vi "bang-bang-ElevatorSim_example.vi"() -> ()   [LabVIEW 2019]
uses:
  <vilib>/Rock Robotics/WPI/ThirdParty/JAS_Junk/TrajLib/Trajectory_Library.lvlib
  <vilib>/Analysis/Matrix/Datatypes/RealMatrix.ctl
  <vilib>/Analysis/Matrix/NI_Matrix.lvlib
  <vilib>/Rock Robotics/WPI/ThirdParty/JAS_Junk/TrajLib/LINEAR_SYSTEM.ctl
  <vilib>/Rock Robotics/WPI/ThirdParty/JAS_Junk/TrajLib/DCMOTOR.CTL
  <vilib>/Rock Robotics/WPI/ThirdParty/JAS_Junk/TrajLib/LINEAR_QUADRATIC_REGULATOR.ctl
  <vilib>/Rock Robotics/WPI/ThirdParty/JAS_Junk/TrajLib/KALMAN_FILTER.ctl
  <vilib>/Rock Robotics/WPI/ThirdParty/JAS_Junk/TrajLib/LINEAR_PLANT_INV_FF.ctl
  <vilib>/Rock Robotics/WPI/ThirdParty/JAS_Junk/TrajLib/LINEAR_SYSTEM_LOOP.ctl
  <vilib>/Rock Robotics/WPI/ThirdParty/JAS_Junk/TrajLib/LINEAR_SYSTEM_SIM.ctl
  <vilib>/Rock Robotics/WPI/ThirdParty/JAS_Junk/TrajLib/ELEVATOR_SIM.ctl
panel:
  in  "Tab Control":T1(tab)
  in  "Turn Motor Off":bool
  in  "Use Bang Bang":bool=TRUE
  out "Battery Voltage":dbl format="%20.3f"
  out "CO Chart":cluster{dbl, "Voltage":dbl}(graph)
  in  "GO UP":bool
  out "Elevator\nHeight \nSetpoint(SP)":dbl(slide) scale=-1.0..6.0
  out "Height":dbl format="%20.3f"
  out "Cor Err":bool
  out "Kalman Filtered\nHeight":dbl format="%20.3f"
  out "PV Chart":T2(graph)
  out "Predict Err":bool
  out "Motor Volt Dmd (CO)":dbl format="%20.3f"
  out "At Top":bool
  out "At Bottom":bool
  out "Motor Amps":dbl format="%20.3f"
  out "Elevator Motor":T3 {"Jr_KgM2" format="%13.5p"; "L_H" format="%13.5p"; "Kt_NMPerAmp" format="%13.5p"; "KvINV_RadPerSecPerVolt" format="%13.5p"; "R_Ohms" format="%13.5p"; "FreeSpeed_RadPerSec" format="%13.5p"; "FreeCurrent_Amps" format="%13.5p"; "StallCurrent_Amps" format="%13.5p"; "StallTorque_NM" format="%13.5p"; "nominalVoltage_Volts" format="%13.5p"}
  out "m_Elevator":T4
  out "Elevator Simulaation":T6 {"GearBox"."Jr_KgM2" format="%13.5p"; "GearBox"."L_H" format="%13.5p"; "GearBox"."Kt_NMPerAmp" format="%13.5p"; "GearBox"."KvINV_RadPerSecPerVolt" format="%13.5p"; "GearBox"."R_Ohms" format="%13.5p"; "GearBox"."FreeSpeed_RadPerSec" format="%13.5p"; "GearBox"."FreeCurrent_Amps" format="%13.5p"; "GearBox"."StallCurrent_Amps" format="%13.5p"; "GearBox"."StallTorque_NM" format="%13.5p"; "GearBox"."nominalVoltage_Volts" format="%13.5p"}
  out "KalmanFilter":T8
  out "Kalman Error":errorcluster
  out "LinearQuadraticRegulator":T9
  out "LQR Error":bool
  out "Linear System Loop":T10
  out "LinSysLoop_Error":bool
  # "THIS IS A SAMPLE  -- THERE ARE BETTER WAYS TO CONTROL THIS OTHER THAN BANG-BANG"
  # "<States,States>"
  # "<States,Inputs>"
  # "<Outputs,States>"
  # "<Outputs,Inputs>"
  # "<States, 1>"
  # "<Outputs, 1>"
  # "<Inputs, 1>"
  # "<Outputs, 1>"
  # "<States,States>"
  # "<States,Inputs>"
  # "<Outputs,States>"
  # "<Outputs,Inputs>"
  # "Steady State Gain  \n<States,Outputs>"
  # "State Estimate <Statess,1>"
  # "<States,States>"
  # "<States,Inputs>"
  # "<Outputs,States>"
  # "<Outputs,Inputs>"
  # "Ref State <States,1>"
  # "Comp and capped \noutput <Inputs,1>"
  # "Controller gain\n<Inputs,States>"
  # "<States,1>"
  # "<FUTURE --- CLAMP TYPE -- For now\nuse Normalize>"
  # "Steady State Gain  \n<States,Outputs>"
  # "State Estimate <Statess,1>"
  # "<States,States>"
  # "<States,Inputs>"
  # "<Outputs,States>"
  # "<Outputs,Inputs>"
  # "<States,1>"
  # "<Inputs,1>"
  # "<States,Inputs>"
  # "<States,States>"
  # "Ref State <States,1>"
  # "Comp and capped \noutput <Inputs,1>"
  # "Controller gain\n<Inputs,States>"
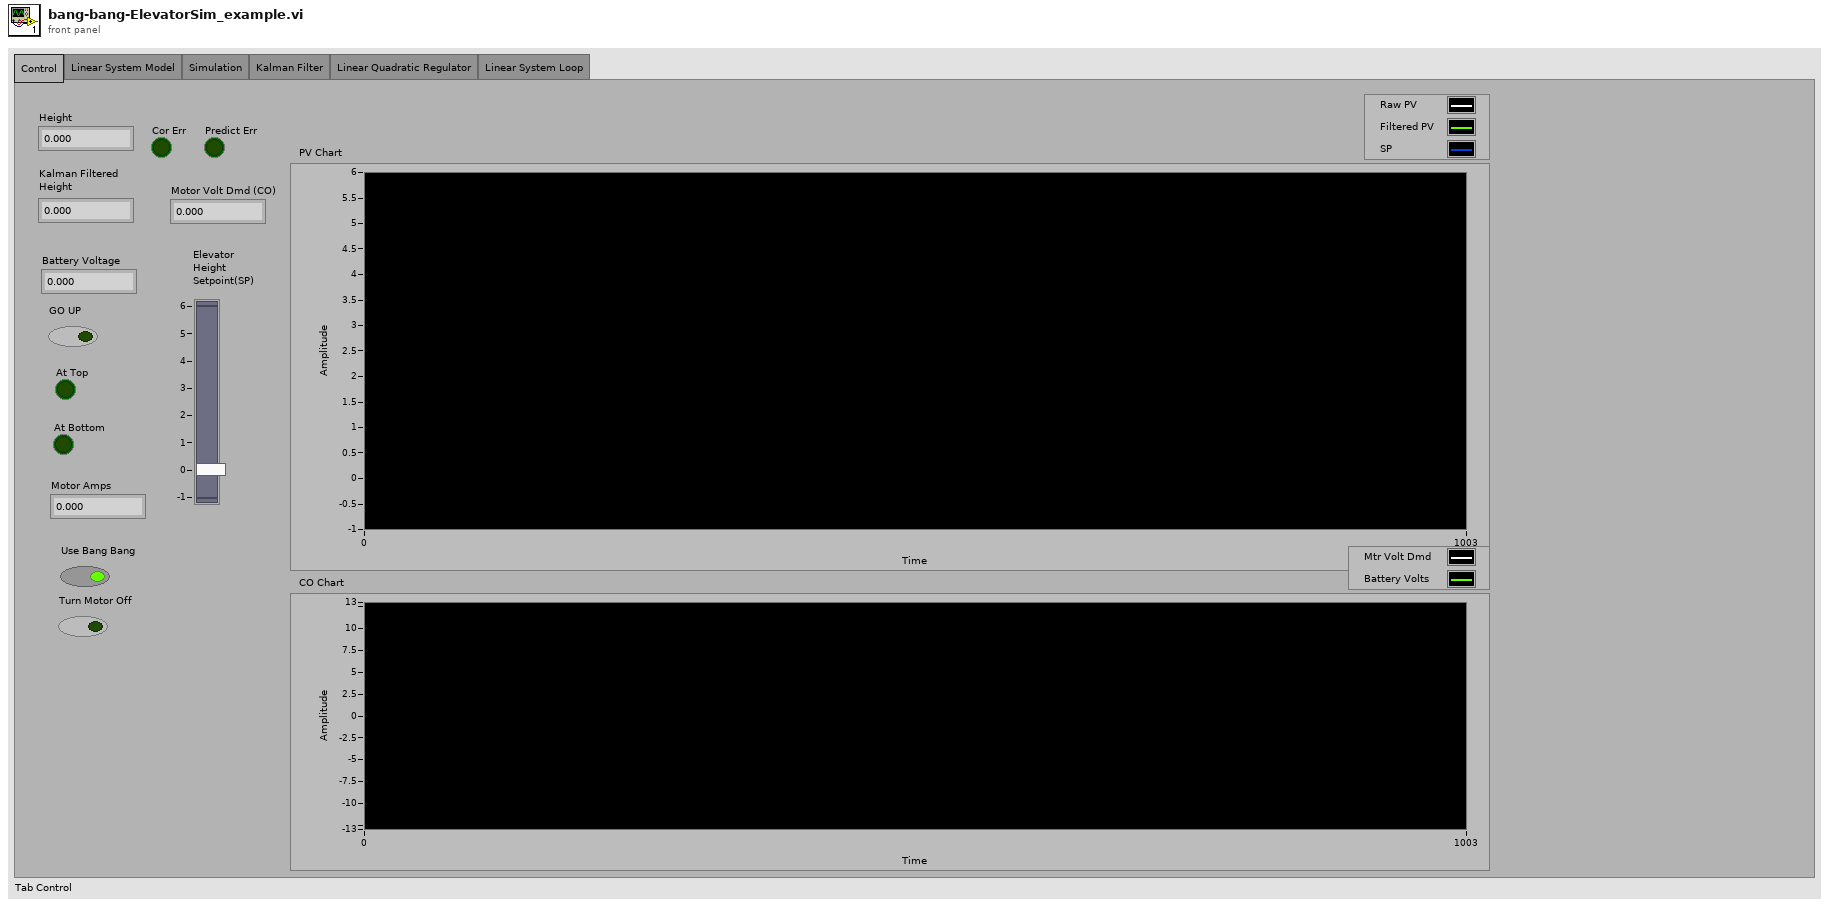
[diagram p1: front panel]
types:
  T1 = enum32{"Control", "Linear System Model", "Simulation", "Kalman Filter", "Linear Quadratic Regulator", "Linear System Loop"}
  T2 = cluster{"upper limit":dbl, "Real Matrix Element":dbl, "Real Matrix Element":dbl}
  T3 = typedef "Trajectory_Library.lvlib/DCMOTOR.CTL" = cluster{"nominalVoltage_Volts":dbl, "StallTorque_NM":dbl, "StallCurrent_Amps":dbl, "FreeCurrent_Amps":dbl, "FreeSpeed_RadPerSec":dbl, "R_Ohms":dbl, "KvINV_RadPerSecPerVolt":dbl, "Kt_NMPerAmp":dbl, "L_H":dbl, "Jr_KgM2":dbl}
  T4 = typedef "Trajectory_Library.lvlib/LINEAR_SYSTEM.ctl" = cluster{"m_A":T5, "m_B":T5, "m_C":T5, "m_D":T5, "States":i32, "Inputs":i32, "Outputs":i32}
  T5 = typedef "NI_Matrix.lvlib/RealMatrix.ctl" = dbl[][]
  T6 = typedef "Trajectory_Library.lvlib/ELEVATOR_SIM.ctl" = cluster{"LinearSystemSim":T7, "GearBox":T3, "Gearing":dbl, "DrumRadius_M":dbl, "MinHeight_M":dbl, "MaxHeight_M":dbl, "CarriageMass_Kg":dbl}
  T7 = typedef "Trajectory_Library.lvlib/LINEAR_SYSTEM_SIM.ctl" = cluster{"m_Plant":T4, "m_X":T5, "m_Y":T5, "m_U":T5, "MeasureStdDev":T5}
  T8 = typedef "Trajectory_Library.lvlib/KALMAN_FILTER.ctl" = cluster{"m_K":T5, "m_xHat":T5, "States":i32, "Outputs":i32, "m_Plant":T4}
  T9 = typedef "Trajectory_Library.lvlib/LINEAR_QUADRATIC_REGULATOR.ctl" = cluster{"m_r":T5, "m_U":T5, "m_K":T5, "States":i32, "Inputs":i32}
  T10 = typedef "Trajectory_Library.lvlib/LINEAR_SYSTEM_LOOP.ctl" = cluster{"Controller":T9, "FeedForward":T11, "Observer":T8, "Next_R":T5, "Clamp Max":T5}
  T11 = typedef "Trajectory_Library.lvlib/LINEAR_PLANT_INV_FF.ctl" = cluster{"m_R":T5, "m_Uff":T5, "m_B":T5, "m_A":T5, "States":i32, "Inputs":i32}
  T12 = cluster{"Position_Meters":dbl, "Real Matrix Element":dbl, "Real Matrix Element":dbl}
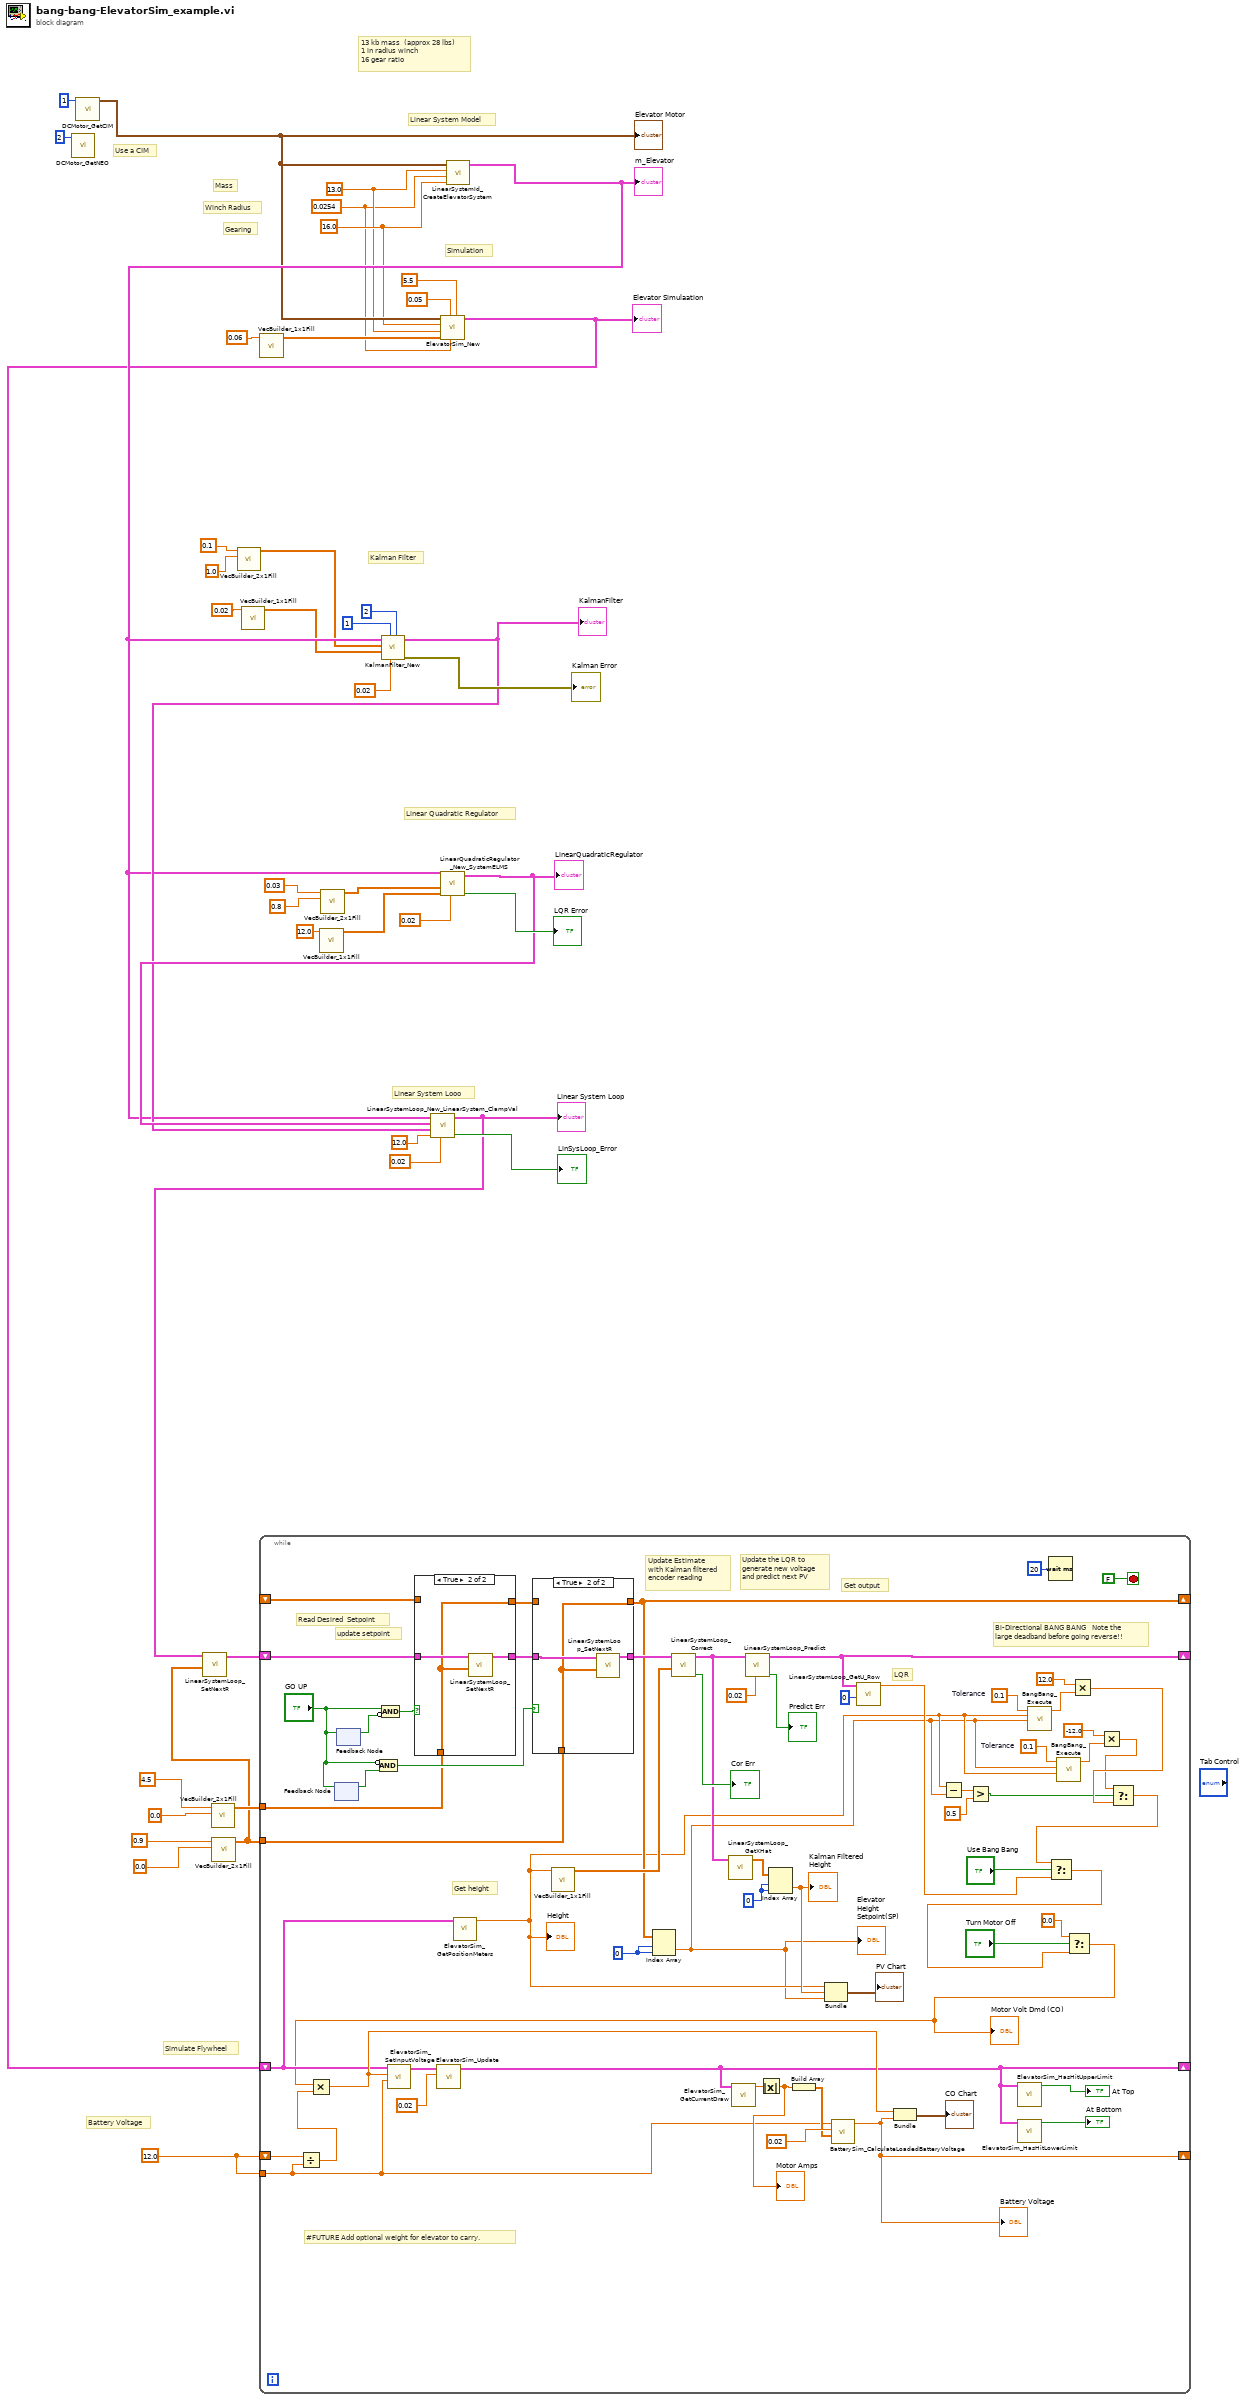
[diagram p0: block diagram]
diagram:
  w26 = 16.0 ("G")
  w24 = 0.0254 ("radiusMeters")
  w25 = 13.0 ("massKg")
  w34 = 12.0
  # "Linear System Looo"
  # "Linear Quadratic Regulator"
  # "Kalman Filter"
  # "Simulation"
  # "Linear System Model"
  # "Mass"
  # "Winch Radius"
  # "Simulate Flywheel"
  # "13 kb mass  (approx 28 lbs)\n1 in radius winch\n16 gear ratio"
  # "Gearing"
  # "Use a CIM"
  # "Battery Voltage"
  n1 = call <vilib>:"DCMotor_GetNEO.vi"("Num Motors"=2) -> ()  [unwired: 10 in, 1 out]
  n2 = call <vilib>:"DCMotor_GetCIM.vi"("Num Motors"=1) -> ("DCMOTOR"=w31:T3)  [unwired: 10 in]
  "Elevator Motor" <- w31
  n3 = call <vilib>:"VecBuilder_2x1Fill.vi"("R1"=0.0, "R0"=4.5 ("RotationsPerMinute")) -> ("output matrix"=w6:T5)  [unwired: 9 in]
  n4 = call <vilib>:"VecBuilder_2x1Fill.vi"("R1"=0.0, "R0"=0.9 ("R0_C0")) -> ("output matrix"=w1:T5)  [unwired: 9 in]
  n5 = call <vilib>:"VecBuilder_2x1Fill.vi"("R1"=1.0, "R0"=0.1 ("R0_C0")) -> ("output matrix"=w17:T5)  [unwired: 9 in]
  n6 = call <vilib>:"VecBuilder_1x1Fill.vi"("R0_C0"=0.02) -> ("output matrix"=w16:T5)  [unwired: 10 in]
  n7 = call <vilib>:"VecBuilder_1x1Fill.vi"("R0_C0"=0.06) -> ("output matrix"=w27:T5)  [unwired: 10 in]
  n8 = call <vilib>:"VecBuilder_1x1Fill.vi"("R0_C0"=12.0) -> ("output matrix"=w10:T5)  [unwired: 10 in]
  n9 = call <vilib>:"VecBuilder_2x1Fill.vi"("R1"=0.8 ("R0_C0"), "R0"=0.03 ("R0_C0")) -> ("output matrix"=w12:T5)  [unwired: 9 in]
  n10 = call <vilib>:"ElevatorSim_New.vi"("MaxHeight_Meters"=5.5, "DrumRadius_Meters"=w24, "MinHeight_Meters"=0.05, "MeasurementStdDev"=w27, "CarriageMass_Kg"=w25, "Gearing"=w26, "GearBox"=w31) -> ("ElevatorSim"=w30:T6)  [unwired: 3 in, 1 out]
  "Elevator Simulaation" <- w30
  n11 = call <vilib>:"LinearSystemId_CreateElevatorSystem.vi"("G"=w26, "radiusMeters"=w24, "massKg"=w25, "DCMOTOR"=w31) -> ("Linearsystem"=w32:T4)  [unwired: 6 in, 1 out]
  "m_Elevator" <- w32
  n12 = call <vilib>:"KalmanFilter_New.vi"("States"=2, "dt_Seconds"=0.02, "Outputs"=1, "MeasurementStdDevs"=w16, "StateStdDevs"=w17, "Plant"=w32) -> ("Error"=→"Kalman Error":errorcluster, "KalmanFilter"=w38:T8)  [unwired: 4 in]
  "KalmanFilter" <- w38
  n13 = call <vilib>:"LinearQuadraticRegulator_New_SystemELMS.vi"("dt_Seconds"=0.02, "Relms"=w10, "Qelms"=w12, "LINEARSYSTEM"=w32) -> ("Error"=→"LQR Error":bool, "LinearQuadraticRegulator"=w39:T9)  [unwired: 6 in]
  "LinearQuadraticRegulator" <- w39
  n14 = call <vilib>:"LinearSystemLoop_New_LinearSystem_ClampVal.vi"("dT_Seconds"=0.02, "Max_Voltage"=12.0, "Observer"=w38, "Controller"=w39, "Plant"=w32) -> ("Error"=→"LinSysLoop_Error":bool, "Linear System Loop"=w2:T10)  [unwired: 5 in]
  "Linear System Loop" <- w2
  n15 = call <vilib>:"LinearSystemLoop_SetNextR.vi"("R"=w1, "input inear System Loop"=w2) -> ("out Linear System Loop"=w3:T10)  [unwired: 8 in, 1 out]
  n16 = while {
    shift-right: [w70] -> _
    shift-left: w3 -> [w98]
    tunnel: w6 -> [w96]
    tunnel: w1 -> [w95]
    shift-right: [w69] -> _
    shift-left: w30 -> [w64]
    shift-right: [w79] -> _
    shift-left: _ -> [w80]
    shift-right: [w72] -> _
    shift-left: w34 -> [w77]
    tunnel: w34 -> [w63]
    stop <- FALSE stop-if-true
    w53 = 0.1  # Tolerance
    w59 = 0.1  # Tolerance
    w78 = 0 ("index (row)")
    w91 = 0 ("index (row)")
    # "Bi-Directional BANG BANG   Note the\nlarge deadband before going reverse!!"
    # "LQR"
    # "Get height"
    # "#FUTURE Add optional weight for elevator to carry."
    # "Get output"
    # "Update the LQR to \ngenerate new voltage\nand predict next PV"
    # "update setpoint"
    # "Read Desired  Setpoint"
    # "Update Estimate\nwith Kalman filtered\nencoder reading"
    n17 = Divide(x=w77, y=w63) -> (x/y=w76:dbl)
    n18 = feedback #1() -> (w102:bool)  [unwired: 1 in]
    n19 = feedback-in #1("GO UP") -> ()
    n20 = feedback-in #2("GO UP") -> ()
    n21 = feedback #2() -> (w103:bool)  [unwired: 1 in]
    n22 = Compound Arithmetic op=AND(invert "GO UP", w102) -> (w99:bool)
    n23 = Compound Arithmetic op=AND("GO UP", invert w103) -> (w100:bool)
    n24 = case shown="True" w100 {
      tunnel: w98 -> [w112 w114]
      tunnel: [w112 w115] -> w97
      tunnel: w96 -> [_ w113]
      tunnel: [w111 w113] -> w81
      tunnel: w80 -> [w111 _]
      frame False {
      }
      frame True {
        n25 = call <vilib>:"LinearSystemLoop_SetNextR.vi"("R"=w113, "input inear System Loop"=w114) -> ("out Linear System Loop"=w115:T10)  [unwired: 8 in, 1 out]
      }
    }
    n26 = call <vilib>:"ElevatorSim_GetPositionMeters.vi"("ElevatorSim"=w64) -> ("Position_Meters"=w50:dbl)  [unwired: 10 in]
    "Height" <- w50
    n27 = case shown="True" w99 {
      tunnel: w97 -> [w107 w109]
      tunnel: [w107 w110] -> w94
      tunnel: w95 -> [_ w108]
      tunnel: w81 -> [w106 _]
      tunnel: [w106 w108] -> w79
      frame False {
      }
      frame True {
        n28 = call <vilib>:"LinearSystemLoop_SetNextR.vi"("R"=w108, "input inear System Loop"=w109) -> ("out Linear System Loop"=w110:T10)  [unwired: 8 in, 1 out]
      }
    }
    n29 = call <vilib>:"VecBuilder_1x1Fill.vi"("R0_C0"=w50) -> ("output matrix"=w93:T5)  [unwired: 10 in]
    n30 = Index Array(array=w79, index (row)=w78, index (col)=w78) -> (element=w49:dbl)
    "Elevator\nHeight \nSetpoint(SP)" <- w49
    n31 = call <vilib>:"LinearSystemLoop_Correct.vi"("Y"=w93, "input inear System Loop"=w94) -> ("Error"=→"Cor Err":bool, "out Linear System Loop"=w87:T10)  [unwired: 8 in]
    n32 = call <vilib>:"LinearSystemLoop_GetXHat.vi"("input inear System Loop"=w87) -> ("XHat"=w90:T5)  [unwired: 10 in]
    n33 = call <vilib>:"LinearSystemLoop_Predict.vi"("dT_Seconds"=0.02, "input inear System Loop"=w87) -> ("Error"=→"Predict Err":bool, "out Linear System Loop"=w70:T10)  [unwired: 8 in]
    n34 = Index Array(array=w90, index (row)=w91, index (col)=w91) -> (element=w89:dbl)
    "Kalman Filtered\nHeight" <- w89
    n35 = Bundle("Position_Meters"=w50, "Real Matrix Element"=w89, "Real Matrix Element"=w49) -> (→"PV Chart":T12)  [unwired: 1 in]
    n36 = call <vilib>:"LinearSystemLoop_GetU_Row.vi"("Row"=0, "input inear System Loop"=w70) -> ("U"=w55:dbl)  [unwired: 9 in]
    n37 = Subtract(x=w50, y=w49) -> (x-y=w48:dbl)
    n38 = Greater?(x=w48, y=0.5) -> (0:w43:bool)
    n39 = call <vilib>:"BangBang_Execute.vi"("Setpoint"=w49, "Measurment"=w50, "Tolerance"=w59) -> ("ControlOutput"=w58:dbl)  [unwired: 6 in, 2 out]
    n40 = Wait (ms)(milliseconds to wait=u32 20) -> ()  [unwired: 1 out]
    n41 = call <vilib>:"BangBang_Execute.vi"("Setpoint"=w50, "Measurment"=w49, "Tolerance"=w53) -> ("ControlOutput"=w52:dbl)  [unwired: 6 in, 2 out]
    n42 = Multiply(x=12.0, y=w58) -> (x*y=w46:dbl)
    n43 = Multiply(x=-12.0, y=w52) -> (x*y=w44:dbl)
    n44 = Select(t=w44, s=w43, f=w46) -> (s? t:f=w45:dbl)
    n45 = Select(t=w45, s="Use Bang Bang", f=w55) -> (s? t:f=w54:dbl)
    n46 = Select(t=0.0, s="Turn Motor Off", f=w54) -> (s? t:f=w60:dbl)
    "Motor Volt Dmd (CO)" <- w60
    n47 = Multiply(x=w60, y=w76) -> (x*y=w71:dbl)
    n48 = call <vilib>:"ElevatorSim_SetInputVoltage.vi"("Battery_Volts"=w63, "Input_Voltage"=w71, "in ElevatorSim"=w64) -> ("out ElevatorSim"=w83:T6)  [unwired: 8 in]
    n49 = call <vilib>:"ElevatorSim_Update.vi"("dT_Seconds"=0.02, "in ElevatorSim"=w83) -> ("out ElevatorSim"=w69:T6)  [unwired: 8 in, 1 out]
    n50 = call <vilib>:"ElevatorSim_GetCurrentDraw.vi"("ElevatorSim"=w69) -> ("Current_Amps"=w66:dbl)  [unwired: 10 in]
    n51 = Absolute Value(x=w66) -> (abs(x)=w65:dbl)
    "Motor Amps" <- w65
    n52 = Build Array(w65) -> (w74:dbl[])
    n53 = call <vilib>:"BatterySim_CalculateLoadedBatteryVoltage.vi"("Currents"=w74, "Resistance_Ohms"=0.02, "NominalVoltage"=w63) -> ("Voltage"=w72:dbl)  [unwired: 8 in]
    "Battery Voltage" <- w72
    n54 = Bundle(w71, "Voltage"=w72) -> (→"CO Chart":cluster{dbl, "Voltage":dbl})  [unwired: 1 in]
    n55 = call <vilib>:"ElevatorSim_HasHitUpperLimit.vi"("ElevatorSim"=w69) -> ("At HIgh LImit"=→"At Top":bool)  [unwired: 10 in]
    n56 = call <vilib>:"ElevatorSim_HasHitLowerLimit.vi"("ElevatorSim"=w69) -> ("AtLowLimit"=→"At Bottom":bool)  [unwired: 10 in]
  }
